vi "Solve1.vi"(8 "Error In":errorcluster, 11 "object in":refnum<class "2021_6.lvclass">) -> (0 "Error Out":errorcluster, 2 "Result":u64, 3 "object out":refnum<class "2021_6.lvclass">)   [LabVIEW 2023, in "2021_6.lvclass"]
uses:
  2021_6.lvclass
  2021_6.lvclass/2021_6.ctl
  7370d572-be9b-4cac-a1ec-f784ae661ada.vi
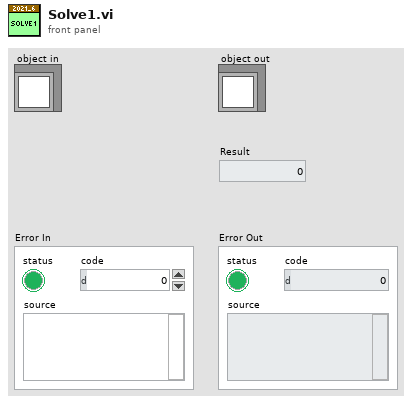
[diagram p1: front panel]
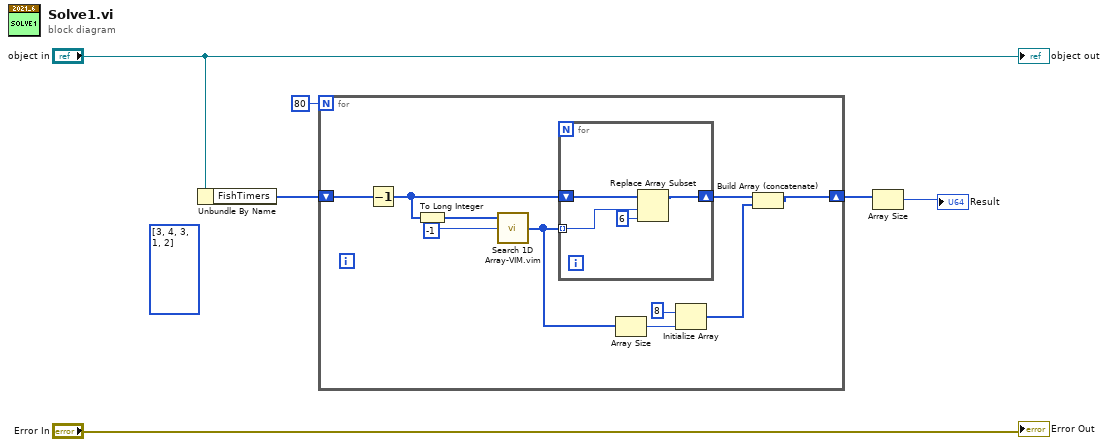
[diagram p0: block diagram]
diagram:
  (unwired) i32[] [3, 4, 3, 1, 2] ("FishTimers")
  n1 = Unbundle By Name("object in") -> ("FishTimers"=w1:i8[])
  n2 = for {
    N: 80 -> [_]
    shift-right: [w11] -> w3
    shift-left: w1 -> [w10]
    n3 = Decrement(x=w10) -> (x-1=w9:i8[])
    n4 = To Long Integer(number=w9) -> (32bit integer=w8:i32[])
    n5 = call "Search 1D Array-VIM.vim"("Array"=w8, "Search Element(s)"=-1) -> ("Indices of Elements"=w16:i32[])  [unwired: 7 in]
    n6 = for {
      shift-right: [w17] -> w13
      shift-left: w9 -> [w20]
      tunnel: w16 -> [w19] mode=indexing
      n7 = Replace Array Subset(array=w20, new element=i8 6 ("new element/subarray"), index=w19) -> (w17:i8[])
    }
    n8 = Array Size(array=w16) -> (size(s)=w15:i32)
    n9 = Initialize Array(i8 8 ("new element/subarray"), w15) -> (w12:i8[])
    n10 = Build Array (concatenate)(w13, w12) -> (w11:i8[])
  }
  n11 = Array Size(array=w3) -> (size(s)=→"Result":i32)
  "Error Out" <- "Error In"
  "object out" <- "object in"
